vi "Inv Kin.vi"(11 "Task Coordinates (cm)":dbl[](array[numeric])) -> (3 "Joint Coordinates (rad)":dbl[](array[numeric]))   [LabVIEW 2018]
panel:
  # "Ex"
  # "Theta 0"
  # "Ey"
  # "Theta 1"
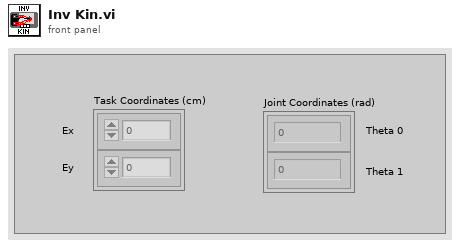
[diagram p1: front panel]
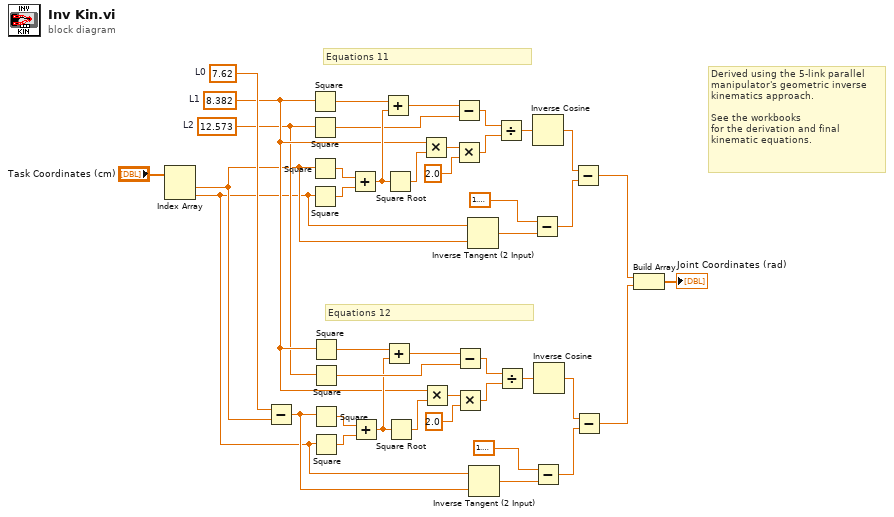
[diagram p0: block diagram]
diagram:
  w9 = 12.573  # L2
  w10 = 8.382  # L1
  w11 = 7.62  # L0
  # "Derived using the 5-link parallel \nmanipulator's geometric inverse \nkinematics approach. \n\nSee the workbooks\nfor the derivation and final\nkinematic equations."
  # "Equations 12"
  # "Equations 11"
  n1 = Index Array(array="Task Coordinates (cm)") -> (element #1=w3:dbl, element #2=w2:dbl)  [unwired: 2 in]
  n2 = Subtract(x=w11, y=w3) -> (x-y=w12:dbl)
  n3 = Square(x=w10) -> (x^2=w39:dbl)
  n4 = Square(x=w9) -> (x^2=w36:dbl)
  n5 = Square(x=w3) -> (x^2=w41:dbl)
  n6 = Square(x=w2) -> (x^2=w42:dbl)
  n7 = Square(x=w10) -> (x^2=w16:dbl)
  n8 = Square(x=w9) -> (x^2=w19:dbl)
  n9 = Square(x=w12) -> (x^2=w14:dbl)
  n10 = Square(x=w2) -> (x^2=w13:dbl)
  n11 = Add(x=w41, y=w42) -> (x+y=w38:dbl)
  n12 = Add(x=w14, y=w13) -> (x+y=w17:dbl)
  n13 = Add(x=w39, y=w38) -> (x+y=w37:dbl)
  n14 = Add(x=w16, y=w17) -> (x+y=w18:dbl)
  n15 = Square Root(x=w38) -> (sqrt(x)=w35:dbl)
  n16 = Square Root(x=w17) -> (sqrt(x)=w20:dbl)
  n17 = Multiply(x=w10, y=w35) -> (x*y=w34:dbl)
  n18 = Multiply(x=w10, y=w20) -> (x*y=w21:dbl)
  n19 = Subtract(x=w37, y=w36) -> (x-y=w32:dbl)
  n20 = Multiply(x=w34, y=2.0) -> (x*y=w31:dbl)
  n21 = Subtract(x=w18, y=w19) -> (x-y=w23:dbl)
  n22 = Multiply(x=w21, y=2.0) -> (x*y=w24:dbl)
  n23 = Inverse Tangent (2 Input)(1:w3, 2:w2) -> (0:w40:dbl)
  n24 = Inverse Tangent (2 Input)(1:w12, 2:w2) -> (0:w15:dbl)
  n25 = Divide(x=w32, y=w31) -> (x/y=w30:dbl)
  n26 = Divide(x=w23, y=w24) -> (x/y=w25:dbl)
  n27 = Subtract(x=1.5707963267948966, y=w40) -> (x-y=w28:dbl)
  n28 = Inverse Cosine(1:w30) -> (0:w29:dbl)
  n29 = Subtract(x=1.5707963267948966, y=w15) -> (x-y=w27:dbl)
  n30 = Inverse Cosine(1:w25) -> (0:w26:dbl)
  n31 = Subtract(x=w29, y=w28) -> (x-y=w6:dbl)
  n32 = Subtract(x=w26, y=w27) -> (x-y=w5:dbl)
  n33 = Build Array(w6, w5) -> (→"Joint Coordinates (rad)":dbl[])
